vi "Untitled 8.vi"() -> ()   [LabVIEW 2019]
uses:
  Generated_client/RPC Messages/Greeter_req.ctl
  Generated_client/RPC Messages/Greeter_req_req_oneof/Greeter_req_req_oneof.lvclass
  Generated_client/RPC Messages/Greeter_res_res_oneof/Greeter_res_res_oneof.lvclass
  Generated_client/RPC Messages/Greeter_MessageA.ctl
  Generated_client/RPC Messages/Greeter_MessageA_oneof_a/Greeter_MessageA_oneof_a.lvclass
  Generated_client/RPC Messages/Greeter_MessageA_oneof_a/Greeter_MessageA_oneof_a.lvclass/Greeter_MessageA_oneof_a.ctl
  Generated_client/RPC Messages/Greeter_req_req_oneof/Greeter_req_req_oneof.lvclass/Greeter_req_req_oneof.ctl
  Generated_client/RPC Messages/Greeter_res_res_oneof/Greeter_res_res_oneof.lvclass/Greeter_res_res_oneof.ctl
  Generated_client/Generated_client.lvlib
panel:
  out "OneOfTemplate out 2":refnum<class "Greeter_MessageA_oneof_a.lvclass">
  out "Get_Val":string
  out "error out 3":errorcluster
  in  "error in (no error) 2":errorcluster
  out "anotherField":string
  in  "Set_Val 2":string
  in  "Set_Val":T1
  out "OneOfTemplate out":refnum<class "Greeter_res_res_oneof.lvclass">
  out "error out 2":errorcluster
  in  "error in (no error)":errorcluster
  out "res_id":i32
  out "error out":errorcluster
  in  "Request Data":T2
  in  "address":string
  in  "error in":errorcluster
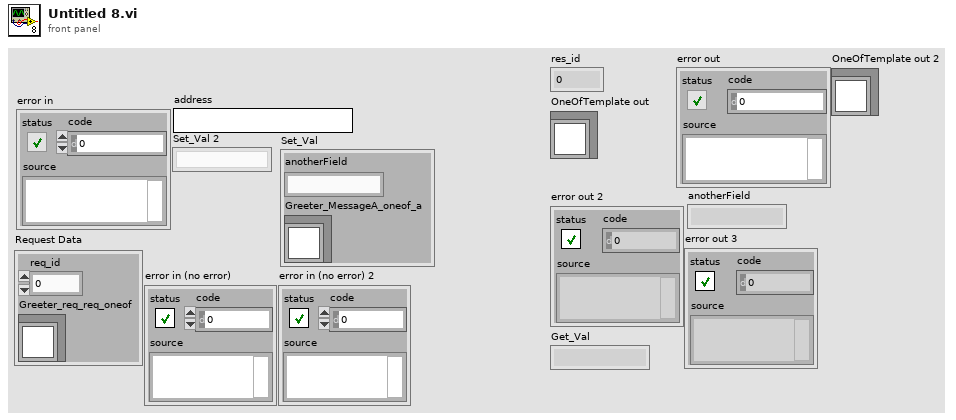
[diagram p1: front panel]
types:
  T1 = typedef "Generated_client.lvlib/Greeter_MessageA.ctl" = cluster{"anotherField":string, "Greeter_MessageA_oneof_a":refnum<class "Greeter_MessageA_oneof_a.lvclass">}
  T2 = typedef "Generated_client.lvlib/Greeter_req.ctl" = cluster{"req_id":i32, "Greeter_req_req_oneof":refnum<class "Greeter_req_req_oneof.lvclass">}
  T3 = typedef "grpc-lvsupport-release.lvlib/grpcId.ctl" = u64
  T4 = typedef "Generated_client.lvlib/Greeter_res.ctl" = cluster{"res_id":i32, "Greeter_res_res_oneof":refnum<class "Greeter_res_res_oneof.lvclass">}
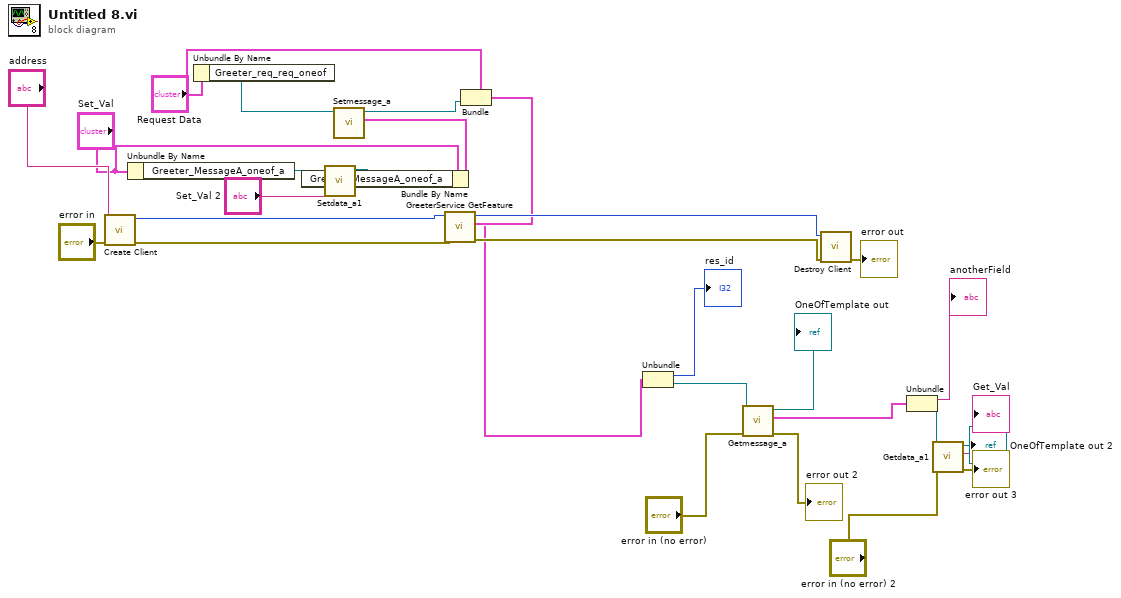
[diagram p0: block diagram]
diagram:
  n1 = call "Create Client.vi"("error in"="error in", "address"="address") -> ("error out"=w27:errorcluster, "gRPC ID Out"=w29:T3)  [unwired: 8 in]
  n2 = Unbundle By Name("Set_Val") -> ("Greeter_MessageA_oneof_a"=w13:refnum<class "Greeter_MessageA_oneof_a.lvclass">)
  n3 = Unbundle By Name("Request Data") -> ("Greeter_req_req_oneof"=w14:refnum<class "Greeter_req_req_oneof.lvclass">)
  n4 = call "Setdata_a1.vi"("Set_Val"="Set_Val 2", "OneOfTemplate in"=w13) -> ("OneOfTemplate out"=w11:refnum<class "Greeter_MessageA_oneof_a.lvclass">)  [unwired: 8 in, 1 out]
  n5 = Bundle By Name(cluster="Set_Val", "Greeter_MessageA_oneof_a"=w11) -> (w9:T1)
  n6 = call "Setmessage_a.vi"("Set_Val"=w9, "OneOfTemplate in"=w14) -> ("OneOfTemplate out"=w8:refnum<class "Greeter_req_req_oneof.lvclass">)  [unwired: 8 in, 1 out]
  n7 = Bundle(cluster="Request Data", "Greeter_req_req_oneof"=w8) -> (w21:T2)  [unwired: 1 in]
  n8 = call "GreeterService GetFeature.vi"("error in"=w27, "Request Data"=w21, "gRPC ID"=w29) -> ("error out"=w26:errorcluster, "Response Data"=w20:T4, "gRPC ID out"=w28:T3)  [unwired: 6 in]
  n9 = Unbundle(w20) -> ("res_id"=→"res_id":i32, "Greeter_res_res_oneof"=w18:refnum<class "Greeter_res_res_oneof.lvclass">)
  n10 = call "Getmessage_a.vi"("error in (no error)"="error in (no error)", "OneOfTemplate in"=w18) -> ("error out"=→"error out 2":errorcluster, "Get_Val"=w7:T1, "OneOfTemplate out"=→"OneOfTemplate out":refnum<class "Greeter_res_res_oneof.lvclass">)  [unwired: 7 in]
  n11 = call "Destroy Client.vi"("error in"=w26, "gRPC ID"=w28) -> ("error out"=→"error out":errorcluster)  [unwired: 9 in]
  n12 = Unbundle(w7) -> ("anotherField"=→"anotherField":string, "Greeter_MessageA_oneof_a"=w5:refnum<class "Greeter_MessageA_oneof_a.lvclass">)
  n13 = call "Getdata_a1.vi"("error in (no error)"="error in (no error) 2", "OneOfTemplate in"=w5) -> ("error out"=→"error out 3":errorcluster, "Get_Val"=→"Get_Val":string, "OneOfTemplate out"=→"OneOfTemplate out 2":refnum<class "Greeter_MessageA_oneof_a.lvclass">)  [unwired: 7 in]
